vi "Send speed logging stop notifier.vi"() -> (0 "error out (No error)":errorcluster)   [LabVIEW 2013]
uses:
  Typedefs/HW config states enum.ctl
  Typedefs/Speed acq notifier data.ctl
  Typedefs/Notifier Function.ctl
  Global Variables/gl_UI Ctrl Refs.vi
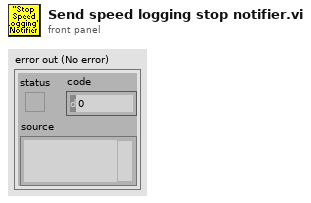
[diagram p1: front panel]
types:
  T1 = typedef "HW config states enum.ctl" = enum16{"Load from file", "Save to file", "Write all", "Read all", "Write XY stage settings", "Write DAQ FPGA settings", "Write Control FPGA settings", "Write Phys Channels", "Clear", "Compare from file"}
  T2 = typedef "Sys Configuration.ctl" = cluster{"XY Stage":T3, "DAQ FPGA":T4, "Control system":T8, "Encoder":T9, "DAQmx Chan":T10, "Computer MAC address":string, "Cam VidRec":T11, "Externalise Triggers":bool, "Laser wavelength (nm)":dbl}
  T3 = typedef "XY Stage config cluster.ctl" = cluster{"COM port":refnum<visa-resource-name>, "XY stage available":bool}
  T4 = typedef "DAQ FPGA config cluster.ctl" = cluster{"Ref":T5, "Target":T6, "Clock Freq (MHz) ":dbl, "input card type":T7, "Samples Wait after Trigger":u16, "AOD fill":u16, "StartupDelay":i32, "Slip Cycle (clock cycles)":u32, "Add Cycle":bool}
  T5 = typedef "FPGA Ref.ctl" = refnum<k20>
  T6 = typedef "nirio_resource_hc.ctl" = tag
  T7 = typedef "FPGA input type AC-DC.ctl" = enum16{"AC Card", "DC Card"}
  T8 = typedef "CTRL system config cluster.ctl" = cluster{"Ethernet opened":bool, "Ethernet Port":u32, "Ctrl FPGA available":bool, "Ctrl FPGA Clock (MHz)":dbl, "Ctrl system MAC address":string, "Control system.Network adapter name":string, "AOD 1 Amplitude":i16, "AOD 2 Amplitude":i16, "AOD 3 Amplitude":i16, "AOD 4 Amplitude":i16, "Data Time Interval (ns)":dbl, "T0 (ns)":dbl, "Ta (ns)":dbl}
  T9 = typedef "Encoder config cluster.ctl" = cluster{"IP address":string, "Port":u16, "Encoder available":bool, "Wheel radius (cm)":dbl}
  T10 = typedef "DAQmx physical channels cluster.ctl" = cluster{"Pockels AO":tag, "Hard shutter AO":tag, "PMT AOs":tag, "Power meter AI":tag}
  T11 = typedef "Cam VidRec HW config setup cluster.ctl" = cluster{"DO flag-Video record":tag, "DO flag-Trial start":tag, "VidRec available":bool}
  T12 = typedef "Notifier Function.ctl" = enum16{"Send notifier", "Wait on notification", "Release notifier"}
  T13 = typedef "Speed acq notifier data.ctl" = cluster{"Log speed data":bool, "File path":path, "Initial timestamp":timestamp}
  T14 = typedef "UI ctrl refs cluster.ctl" = cluster{"Top level VI path":path, "Top level VI ref":refnum<vi>, "User menu ref":refnum<k9>, "Sub Panel control":refnum<vi>, "Imaging Param Tab":refnum<vi>, "Occurrence-Start drivers":refnum<k4>, "Occurrence-Speed logging initialised":refnum<k4>, "Occurrence-XYZ stage initialised":refnum<k4>, "Exit button":refnum<vi>, "Status ind":refnum<vi>, "Return to Origin":refnum<vi>, "Speed Logging":refnum<vi>, "Time Lapse":refnum<vi>, "Live Imaging":refnum<vi>, "AOL Z Stack":refnum<vi>, "Motor Z Stack":refnum<vi>, "Funct Acq button":refnum<vi>, "Hard Shutter":refnum<vi>, "Virtual Shutter":refnum<vi>, "Laser Power":refnum<vi>, "AOL Mode":refnum<vi>, "Frame Size":refnum<vi>, "Field of View":refnum<vi>, "Dwell Time":refnum<vi>, "Zoom":refnum<vi>, "AOL Z":refnum<vi>, "Objective":refnum<vi>, "Axis":refnum<vi>, "Paths & Names":refnum<vi>, "Experiment folder path (ind.)":refnum<vi>, "Last State (Ind.)":refnum<vi>, "Laser wavelength ind (nm)":refnum<vi>, "Averages":refnum<vi>, "Angle (degrees)":refnum<vi>, "X centre":refnum<vi>, "Y centre":refnum<vi>, "Plane Mode":refnum<vi>, "# Planes":refnum<vi>, "Z Start":refnum<vi>, "Z Stop":refnum<vi>, "Z Step":refnum<vi>, "PMT 1":refnum<vi>, "PMT 2":refnum<vi>, "Stage XYZ Position":refnum<vi>, "Pockels@Z Start":refnum<vi>, "Pockels@Z Stop":refnum<vi>, "Obtain Z Start":refnum<vi>, "Obtain Z Stop":refnum<vi>, "Live stim.trig.period":refnum<vi>, "Live stim.trig.enable":refnum<vi>, "Funct. Acq. Pockels Modulation":refnum<vi>, "Enable Video Recording":refnum<vi>, "Video Record-Live Imaging":refnum<vi>, "Video Record-Funct acq":refnum<vi>, "AOL Z-stack Chirps Ready (ind)":refnum<vi>, "Center freq ind (nm)":refnum<vi>, "Logging queue (ind)":refnum<vi>, "Back aperture power (ind.)":refnum<vi>, "Power after objective (ind.)":refnum<vi>, "Switch user":refnum<vi>}
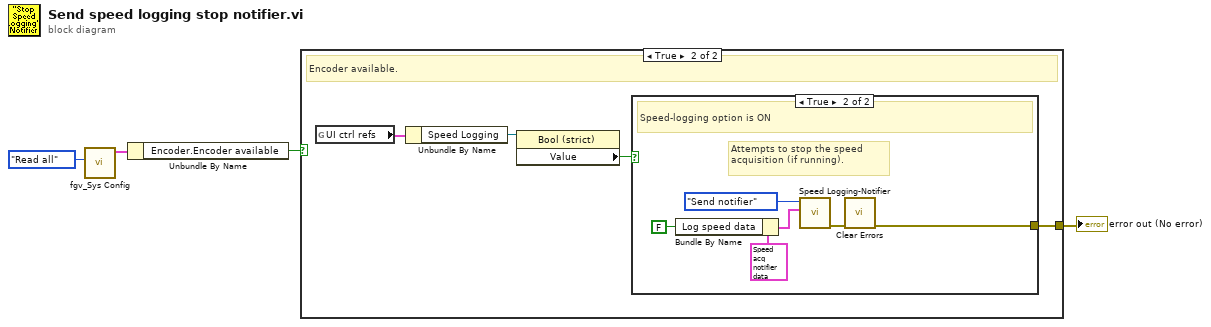
[diagram p0: block diagram]
diagram:
  n1 = call "fgv_Sys Config.vi"("Function"=HW_config_states_enum."Read all") -> ("System Config out"=w4:T2)  [unwired: 9 in, 1 out]
  n2 = Unbundle By Name(w4) -> ("Encoder.Encoder available"=w2:bool)
  n3 = case shown="True" w2 {
    tunnel: [_ w5] -> w1
    frame False {
      # "Encoder unavailable"
    }
    frame True {
      # "Encoder available."
      n4 = global read "gl_UI Ctrl Refs.vi" "UI ctrl refs"() -> (w6:T14)
      n5 = Unbundle By Name(w6) -> ("Speed Logging"=w8:refnum<vi>)
      n6 = property class="Bool (strict)"(reference=w8) -> ("Value"=w7:bool)  [unwired: 1 in, 2 out]
      n7 = case shown="True" w7 {
        tunnel: [_ w9] -> w5
        frame False {
        }
        frame True {
          # "Attempts to stop the speed acquisition (if running)."
          # "Speed-logging option is ON"
          n8 = Bundle By Name(cluster=T13 {"Log speed data"=TRUE, "File path"=path "", "Initial timestamp"=timestamp(0 s since 1904-01-01)} ("Value to send"), "Log speed data"=FALSE ("Log?")) -> (w11:T13)
          n9 = call "Speed Logging-Notifier.vi"("Value to send"=w11, "Notifier Function"=Notifier_Function."Send notifier") -> ("error out"=w10:errorcluster)  [unwired: 7 in, 2 out]
          n10 = call <vilib>:"Clear Errors.vi"("error in (no error)"=w10) -> ("error out"=w9:errorcluster)  [unwired: 6 in]
        }
      }
    }
  }
  "error out (No error)" <- w1
